vi "Get Port.vi"(8 "error in (no error)":errorcluster caption="entrée d'erreur (pas d'erreur)", 11 "Class DIO en entrée":refnum<class "Class Instrument DIO.lvclass">) -> (0 "error out":errorcluster caption="sortie d'erreur", 2 "Port":u8, 3 "Class DIO en Sortie":refnum<class "Class Instrument DIO.lvclass">)   [LabVIEW 2020, in "Library Instrument & Equipement.lvlib" / "Library Instruments.lvlib" / "Class Instrument DIO.lvclass"]
uses:
  Class Instrument DIO.lvclass
  Class Instrument DIO.lvclass/Class Instrument DIO.ctl
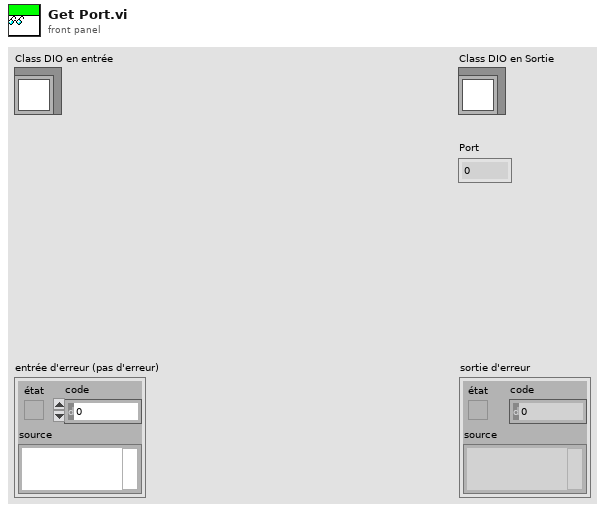
[diagram p1: front panel]
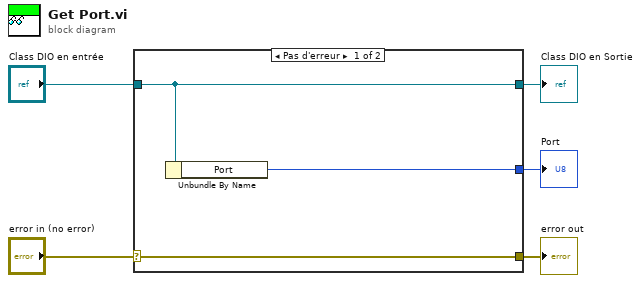
[diagram p0: block diagram]
diagram:
  n1 = case shown="Pas d'erreur" "error in (no error)" {
    selector: "error in (no error)" -> [w8 w9]
    tunnel: [w8 w9] -> w4
    tunnel: [w7 w10] -> w2
    tunnel: "Class DIO en entrée" -> [w7 w10]
    tunnel: [w6 _] -> w1
    frame No Error {
      n2 = Unbundle By Name(w7) -> ("Port"=w6:u8)
    }
    frame Error {
    }
  }
  "error out" <- w4
  "Class DIO en Sortie" <- w2
  "Port" <- w1
